vi "AUTON_Init.vi"(11 "Default File":i32) -> (0 "Auton Array":dbl[][](array[numeric]) format="%0.3f", 2 "Auton Files":string[](array[string]), 3 "Number of Auton Files":i64)   [LabVIEW 2013]
uses:
  <vilib>/Rock Robotics/WPI/DriverStation/DriverStationLCD/WPI_DriverStationLCDLCDLine.ctl
  <vilib>/Utility/file.llb/Read From Spreadsheet File (DBL).vi
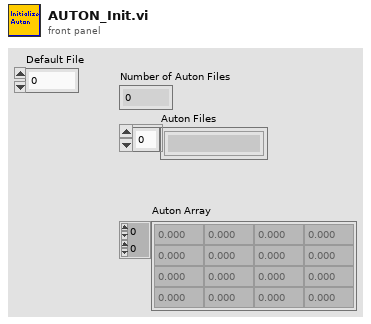
[diagram p1: front panel]
types:
  T1 = typedef "WPI_DriverStationLCDLCDLine.ctl" = enum16{"Main - Line 1", "User - Line 2", "User - Line 3", "User - Line 4", "User - Line 5", "User - Line 6"}
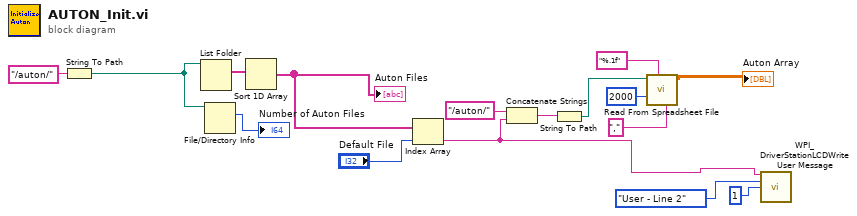
[diagram p0: block diagram]
diagram:
  n1 = String To Path(string="/auton/") -> (path=w5:path)
  n2 = List Folder(path=w5) -> (filenames=w6:string[])  [unwired: 1 in, 5 out]
  n3 = File/Directory Info(path=w5) -> (size=→"Number of Auton Files":i64)  [unwired: 1 in, 6 out]
  n4 = Sort 1D Array(array=w6) -> (sorted array=w8:string[])
  "Auton Files" <- w8
  n5 = Index Array(array=w8, index="Default File") -> (element=w2:string)
  n6 = Concatenate Strings("/auton/" ("string"), w2) -> (w13:string)
  n7 = String To Path(string=w13) -> (path=w12:path)
  n8 = call-poly <vilib>:"Read From Spreadsheet File.vi"("delimiter (\\t)"="," ("delimiter (\\t)"), "format (%.3f)"="%.1f", "number of rows (all:-1)"=2000, "file path (dialog if empty)"=w12) -> ("all rows"=→"Auton Array":dbl[][])  [unwired: 1 in, 6 out]
  n9 = call <vilib>:"WPI_DriverStationLCDWrite User Message.vi"("line text"=w2, "line"=WPI_DriverStationLCDLCDLine."User - Line 2", "starting column"=i8 1) -> ()  [unwired: 2 in, 11 out]
